vi "Set Clock (Calendar).vi"(0 "VISA resource name":refnum<visa-resource-name>, 1 "Minute (0)":i32, 2 "Hour (0)":i32, 5 "Second (0)":i32, 7 "Day (1)":i32=1, 9 "Month (1: January)":u32(ring)=1 items=["", "January", "February", "March", "April", "May", "June", "July", "August", "Septemeber", "October", "Novemeber", "December"], 11 "error in (no error)":errorcluster, 12 "Year (2002)":i32=2002) -> (4 "VISA resource name out":refnum<visa-resource-name>, 15 "error out":errorcluster)   [LabVIEW 2011, in "Fluke 5XXX Series Multicalibrators.lvlib"]
doc: "This VI configures the instrument's internal clock and calendar.\n\nNotes:\n\n(1) This VI is available only for instrument models 5520A, 5700A and 5720A.\n\n(2) You will be unable to set the clock (calendar) if the rear panel CALIBRATION switch is in the ENABLE position."
uses:
  Fluke 5XXX Series Multicalibrators.lvlib
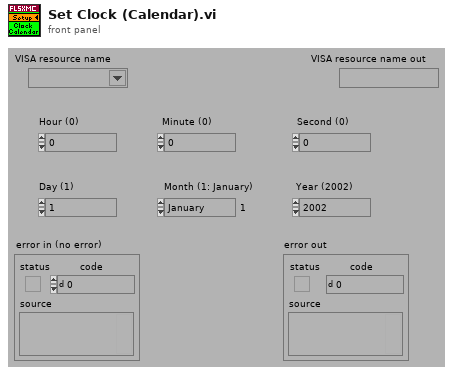
[diagram p1: front panel]
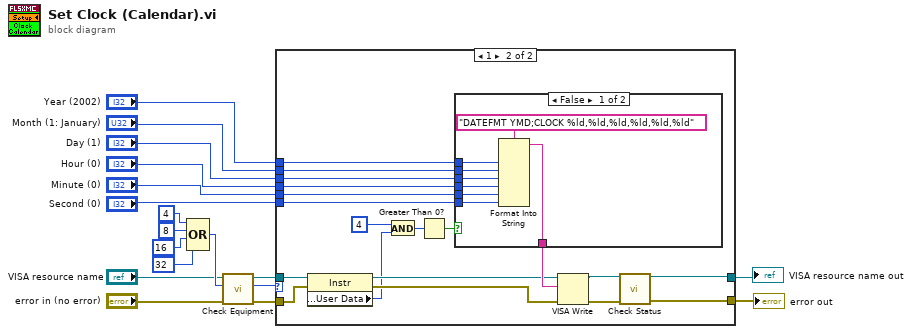
[diagram p0: block diagram]
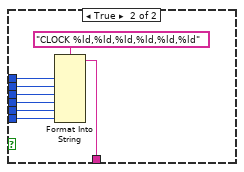
[diagram p3: hidden frame]
diagram:
  n1 = Compound Arithmetic op=OR(4 ("Numeric"), 8 ("Numeric"), 16 ("Numeric"), 32 ("Numeric")) -> (w12:i32)
  n2 = call "Check Equipment.vi"("error in (no error)"="error in (no error)", "Bit Mask"=w12, "VISA resource name"="VISA resource name") -> ("error out"=w15:errorcluster, "Present?"=w13:u32, "VISA resource name out"=w14:refnum<visa-resource-name>)  [unwired: 6 in]
  n3 = case shown="1" w13 {
    tunnel: [w19 w36] -> w10
    tunnel: w15 -> [w20 w26]
    tunnel: w14 -> [w19 w28]
    tunnel: [w20 w39] -> w11
    tunnel: "Year (2002)" -> [_ w34]
    tunnel: "Month (1: January)" -> [_ w33]
    tunnel: "Day (1)" -> [_ w32]
    tunnel: "Hour (0)" -> [_ w31]
    tunnel: "Minute (0)" -> [_ w30]
    tunnel: "Second (0)" -> [_ w29]
    frame 0, Default {
    }
    frame 1 {
      n4 = property class="Instr"(reference=w28, error in=w26) -> (reference out=w27:refnum<visa-resource-name>, error out=w25:errorcluster, "General Settings:User Data"=w24:u32)
      n5 = And(x=u32 4 ("Numeric"), y=w24) -> (x .and. y?=w22:u32)
      n6 = Greater Than 0?(x=w22) -> (x > 0?=w21:bool)
      n7 = case shown="False" w21 {
        tunnel: [w46 w54] -> w35
        tunnel: w34 -> [w45 w53]
        tunnel: w33 -> [w44 w52]
        tunnel: w32 -> [w43 w51]
        tunnel: w31 -> [w42 w50]
        tunnel: w30 -> [w41 w49]
        tunnel: w29 -> [w40 w48]
        frame False {
          n8 = Format Into String(format string="DATEFMT YMD;CLOCK %ld,%ld,%ld,%ld,%ld,%ld", w45, w44, w43, w42, w41, w40) -> (resulting string=w46:string)  [unwired: 2 in, 1 out]
        }
        frame True {
          n9 = Format Into String(format string="CLOCK %ld,%ld,%ld,%ld,%ld,%ld", w53, w52, w51, w50, w49, w48) -> (resulting string=w54:string)  [unwired: 2 in, 1 out]
        }
      }
      n10 = VISA Write(VISA resource name=w27, write buffer=w35, error in (no error)=w25) -> (VISA resource name out=w37:refnum<visa-resource-name>, error out=w38:errorcluster)  [unwired: 1 out]
      n11 = call "Check Status.vi"("VISA resource name"=w37, "error in (no error)"=w38) -> ("VISA resource name out"=w36:refnum<visa-resource-name>, "error out"=w39:errorcluster)  [unwired: 12 in]
    }
  }
  "VISA resource name out" <- w10
  "error out" <- w11
